vi "User Event-Settings-Value Change.vi"(8 "Error In":errorcluster, 11 "Appearance Actor in":refnum<class "Appearance Actor.lvclass">) -> (0 "Error Out":errorcluster, 3 "Appearance Actor out":refnum<class "Appearance Actor.lvclass">)   [LabVIEW 2021, in "Appearance Actor.lvlib" / "Appearance Actor.lvclass"]
doc: "Handles Settings Event. By Default, do nothing. Override this method to change its behavior."
uses:
  Appearance Actor.lvclass
  Appearance Actor.lvclass/Appearance Actor.ctl
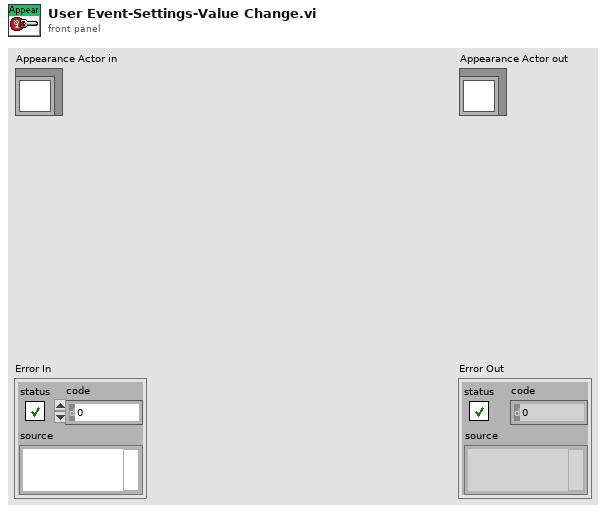
[diagram p1: front panel]
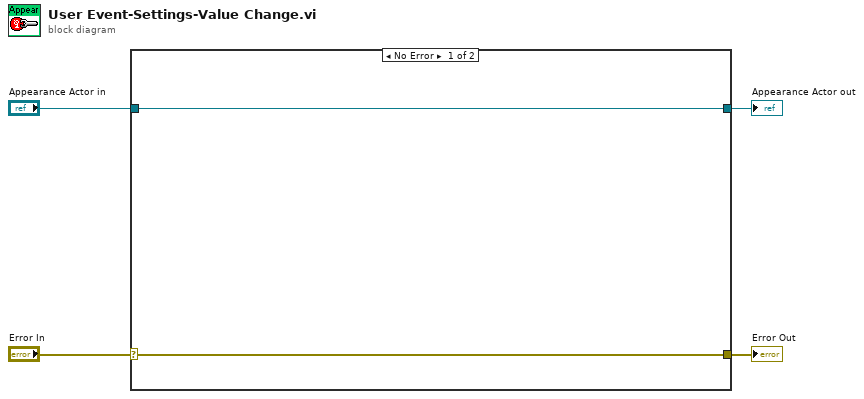
[diagram p0: block diagram]
diagram:
  n1 = case shown="No Error" "Error In" {
    selector: "Error In" -> [w5 w8]
    tunnel: [w5 w8] -> w3
    tunnel: [w6 w7] -> w1
    tunnel: "Appearance Actor in" -> [w6 w7]
    frame No Error {
    }
    frame Error {
    }
  }
  "Error Out" <- w3
  "Appearance Actor out" <- w1
